vi "Remove Entity.vi"(8 "error in (no error)":errorcluster, 10 "Conditum:Entity":refnum<class "Entity.lvclass">, 11 "Entity Collection in":refnum<class "Entity Collection.lvclass">) -> (0 "error out":errorcluster, 3 "Entity Collection out":refnum<class "Entity Collection.lvclass">)   [LabVIEW 2020, in "Conditu2.lvlib" / "Columns.lvlib" / "Entity Collection.lvclass"]
uses:
  Entity Collection.lvclass
  Entity/Entity.lvclass
  Entity/Entity.lvclass/Entity.ctl
  ID/ID.lvclass/ID.ctl
  Entity Collection.lvclass/Entity Collection.ctl
  ID/Get.vi
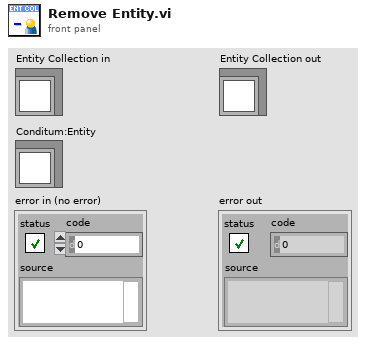
[diagram p1: front panel]
types:
  T1 = typedef "Conditu2.lvlib/Entity ID.ctl" = i64
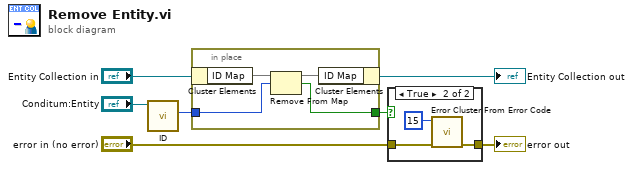
[diagram p0: block diagram]
diagram:
  n1 = call "ID.vi"("Entity in"="Conditum:Entity") -> ("ID"=w5:T1)  [unwired: 9 in, 1 out]
  n2 = in-place {
    in-place-border: w5 -> [w10]
    in-place-border: [w8] -> w2
    n3 = in-place-cluster #1("Entity Collection in") -> ("ID Map"=w11:map{T1, i32})
    n4 = Remove From Map(10:w10, 11:w11) -> (2:w8:bool, 3:w9:map{T1, i32})  [unwired: 1 out]
    n5 = in-place-cluster #1("ID Map"=w9) -> (→"Entity Collection out":refnum<class "Entity Collection.lvclass">)
  }
  n6 = case shown="True" w2 {
    tunnel: "error in (no error)" -> [w12 w15]
    tunnel: [w12 w13] -> w1
    frame False {
    }
    frame True {
      n7 = call <vilib>:"Error Cluster From Error Code.vi"("error in (no error)"=w15, "error code (0)"=15) -> ("error out"=w13:errorcluster)  [unwired: 7 in]
    }
  }
  "error out" <- w1
